vi "Pcre2GetMatchOffsetsFromOvector8.vi"(8 "error in":errorcluster, 9 "OvectorCount":u32, 10 "OvectorSize":u64, 11 "pOvector":u64 format="%.0x") -> (0 "error out":errorcluster, 1 "OffsetsPastMatch":i32[](array[numeric]), 2 "MatchOffsets":i32[](array[numeric]), 3 "pOvector":u64 format="%.0x")   [LabVIEW 2021, in "libpcre2-8.lvlib"]
uses:
  libpcre2-8.lvlib
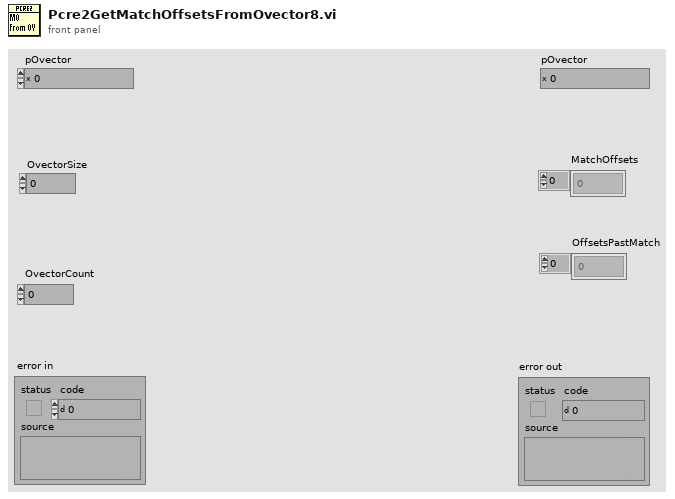
[diagram p1: front panel]
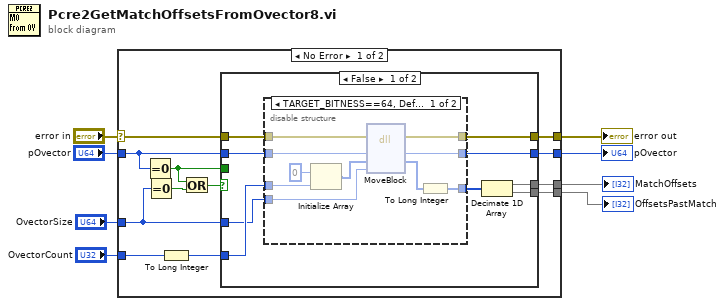
[diagram p0: block diagram]
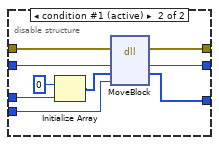
[diagram p2: hidden frame]
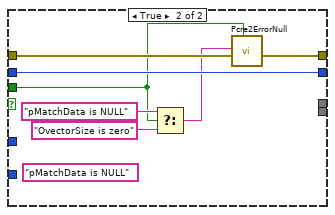
[diagram p3: hidden frame]
diagram:
  n1 = case shown="No Error" "error in" {
    selector: "error in" -> [w10 w57]
    tunnel: [w20 w57] -> w8
    tunnel: [w19 w56] -> w7
    tunnel: "OvectorCount" -> [w17 _]
    tunnel: "OvectorSize" -> [w14 _]
    tunnel: "pOvector" -> [w13 w56]
    tunnel: [w12 _] -> w3
    tunnel: [w11 _] -> w2
    frame No Error {
      n2 = Equal To 0?(x=w13) -> (x = 0?=w9:bool)
      n3 = Equal To 0?(x=w14) -> (x = 0?=w16:bool)
      n4 = To Long Integer(number=w17) -> (32bit integer=w15:i32)
      n5 = Or(x=w9, y=w16) -> (x .or. y?=w18:bool)
      n6 = case shown="False" w18 {
        tunnel: w10 -> [w29 w52]
        tunnel: [w25 w51] -> w20
        tunnel: w13 -> [w28 w55]
        tunnel: [w24 w55] -> w19
        tunnel: w15 -> [w27 _]
        tunnel: w14 -> [w26 _]
        tunnel: [w22 _] -> w12
        tunnel: [w21 _] -> w11
        tunnel: w9 -> [_ w49]
        frame False {
          n7 = disable-structure shown="TARGET_BITNESS==64, Default" {
            disable-tunnel: w28 -> [w39 w48]
            disable-tunnel: [w38 w47] -> w24
            disable-tunnel: [w37 w46] -> w25
            disable-tunnel: w29 -> [w36 w45]
            disable-tunnel: w26 -> [w34 w43]
            disable-tunnel: w27 -> [w33 w42]
            disable-tunnel: [w30 w40] -> w23
            frame condition #0 {
              n8 = Initialize Array(i64 0 ("element"), w33) -> (w32:i64[])
              n9 = dll-call lib="LabVIEW" fn="MoveBlock"(error in=w36, "pointerSrc"=w39, "pointerDest"=w32, "size"=w34) -> (error out=w37:errorcluster, "pointerSrc"=w38:u64, "pointerDest"=w31:i64[])  [unwired: 4 in, 1 out]
              n10 = To Long Integer(number=w31) -> (32bit integer=w30:i32[])
            }
            frame condition #1 (active) {
              n11 = Initialize Array(0 ("element"), w42) -> (w41:i32[])
              n12 = dll-call lib="LabVIEW" fn="MoveBlock"(error in=w45, "pointerSrc"=w48, "pointerDest"=w41, "size"=w43) -> (error out=w46:errorcluster, "pointerSrc"=w47:u64, "pointerDest"=w40:i32[])  [unwired: 4 in, 1 out]
            }
          }
          n13 = Decimate 1D Array(w23) -> (w22:i32[], w21:i32[])
        }
        frame True {
          (unwired) "pMatchData is NULL"
          n14 = Select(t="pMatchData is NULL", s=w49, f="OvectorSize is zero") -> (s? t:f=w50:string)
          n15 = call "Pcre2ErrorNull.vi"("IsPointer? (F)"=w49, "error in"=w52, "What"=w50) -> ("error out"=w51:errorcluster)  [unwired: 8 in]
        }
      }
    }
    frame Error {
    }
  }
  "pOvector" <- w7
  "error out" <- w8
  "MatchOffsets" <- w3
  "OffsetsPastMatch" <- w2
